vi "Main.vi"() -> ()   [LabVIEW 2017]
uses:
  TypeDefs/StateMachnie_States.ctl
  <vilib>/ni845x/ni845x.llb/ni845xI2cConfiguration.ctl
  <vilib>/ni845x/ni845x.llb/ni845xControl.ctl
  TypeDefs/AD5933_Config.ctl
  TypeDefs/MeasurementConfig.ctl
  TypeDefs/MeasurementRawData.ctl
  TypeDefs/AD5933_OperationState.ctl
  <vilib>/ni845x/ni845x.llb/NI-845x I2C Close Configuration Reference.vi
  <vilib>/ni845x/ni845x.llb/NI-845x Close Device Reference.vi
  GlobalVariables/Delimiter.vi
  GlobalVariables/MeasurementCluster.vi
  <vilib>/imath/engines/lvmath2/RunTimeEngine/Managers/WorkSpace/UID Generator.vi
  <vilib>/imath/engines/lvmath2/RunTimeEngine/ArithmeticOperatorToken/NIMS_ArithmeticOperator_plus.vi
  <instcachedir>/0/NIMS_ArithmeticOperator_plus_9255C7DA94A9479C92F91DC2DA9A664F.lvgen/NIMS_ArithmeticOperator_plus_9255C7DA94A9479C92F91DC2DA9A664F_004.vi
  <vilib>/imathl/engines/lvmath/Functions/Error Handling/Create Error.vi
  <vilib>/imath/engines/lvmath2/RunTimeEngine/ArithmeticOperatorToken/NIMS_ArithmeticOperator_rightdiv.vi
  <instcachedir>/0/NIMS_ArithmeticOperator_rightdiv_EFA95513F40C4B3084B27C9DE6D5A167.lvgen/NIMS_ArithmeticOperator_rightdiv_EFA95513F40C4B3084B27C9DE6D5A167_005.vi
  <vilib>/imath/engines/lvmath2/RunTimeEngine/RunTimeType/NIMS_RunTimeType_From StrictType (excl LVString).vi
  <instcachedir>/0/NIMS_RunTimeType_From StrictType (excl LVString)_1019F277F0A747EDBCA0F6C52CA54500.lvgen/NIMS_RunTimeType_From StrictType (excl LVString)_1019F277F0A747EDBCA0F6C52CA54500_000.vi
  <vilib>/imath/engines/lvmath2/RunTimeEngine/LocalVariableDefStatement/MC_LocalVariableDefStatement_Display.vi
  <vilib>/imath/engines/lvmath2/RunTimeEngine/Managers/SymbolTable/Clear UID.vi
  <vilib>/imath/engines/lvmath2/RunTimeEngine/NodeEndStatement/NIMS_NodeEndStatement_Output.vi
  <instcachedir>/0/NIMS_NodeEndStatement_Output_53EC0D466D134D7ABD903AC30B43404B.lvgen/NIMS_NodeEndStatement_Output_53EC0D466D134D7ABD903AC30B43404B_005.vi
  <vilib>/imath/engines/lvmath2/RunTimeEngine/ErrorHandling/NIMS_Finalize Error.vi
  <vilib>/imath/engines/lvmath2/RunTimeEngine/Managers/SymbolTable/NIMS_WorkSpace.lvlib
panel:
  out "|Z|,phi vs Time (old)":cluster{"X":dbl, "Y":dbl, "X 2":dbl}[](graph)
  out "Temperature vs Time (old)":cluster{"x-y":dbl, "Temperature":dbl}[](graph)
  out "Real,Imag vs Frequency (old)":cluster{"X":dbl, "Y":dbl, "X 2":dbl}[](graph)
  out "Measurement Indicator":bool
  out "|Z|,phi vs Frequency (old)":cluster{dbl, "Impedance":dbl, "Phase":dbl}[](graph)
  in  "Calibrate":bool
  in  "Ref. Resistor":dbl=100000.0 format="%#_13p"
  in  "Start":bool
  in  "Set Configuration":bool
  in  "Stop Measurement":bool
  out "Next measurement":dbl
  in  "Stop Updating Frequeny Plot":bool
  in  "Tab Control":T1(tab)
  out "|Z|,phi vs Frequency":cluster{dbl, "Impedance":dbl, "Phase":dbl}[](graph) caption="XY Graph"
  out "Real,Imag vs Frequency":cluster{dbl, "Impedance":dbl, "Phase":dbl}[](graph) caption="XY Graph"
  out "Temperature vs Time":cluster{"x-y":dbl, "Temperature":dbl}[](graph) caption="XY Graph"
  in  "Frequency [Hz]":dbl(slide) min=5000.0 max=100000.0 step=2500.0 scale=5000.0..100000.0 scale format="%#_6p"
  out "|Z|,phi vs Time":cluster{dbl, "Impedance":dbl, "Phase":dbl}[](graph) caption="XY Graph"
  # "FEHLER Suche:\n- Bei Messung mit 100k Widerstand\n    - Hohe schwankungen zwischen Inf und 0 (Magnitde)\n    - Wenn dann ist Imag Wert sehr hoch, Real recht klein !?!\n       - Sollte umgekehrt Re hocher Leitwert, Im geringer Wert"
  # "Mehrere Werte mitteln ?\nGain Faktor Messen\nAbspeichern noch nicht implementiert!"
  # "[s]"
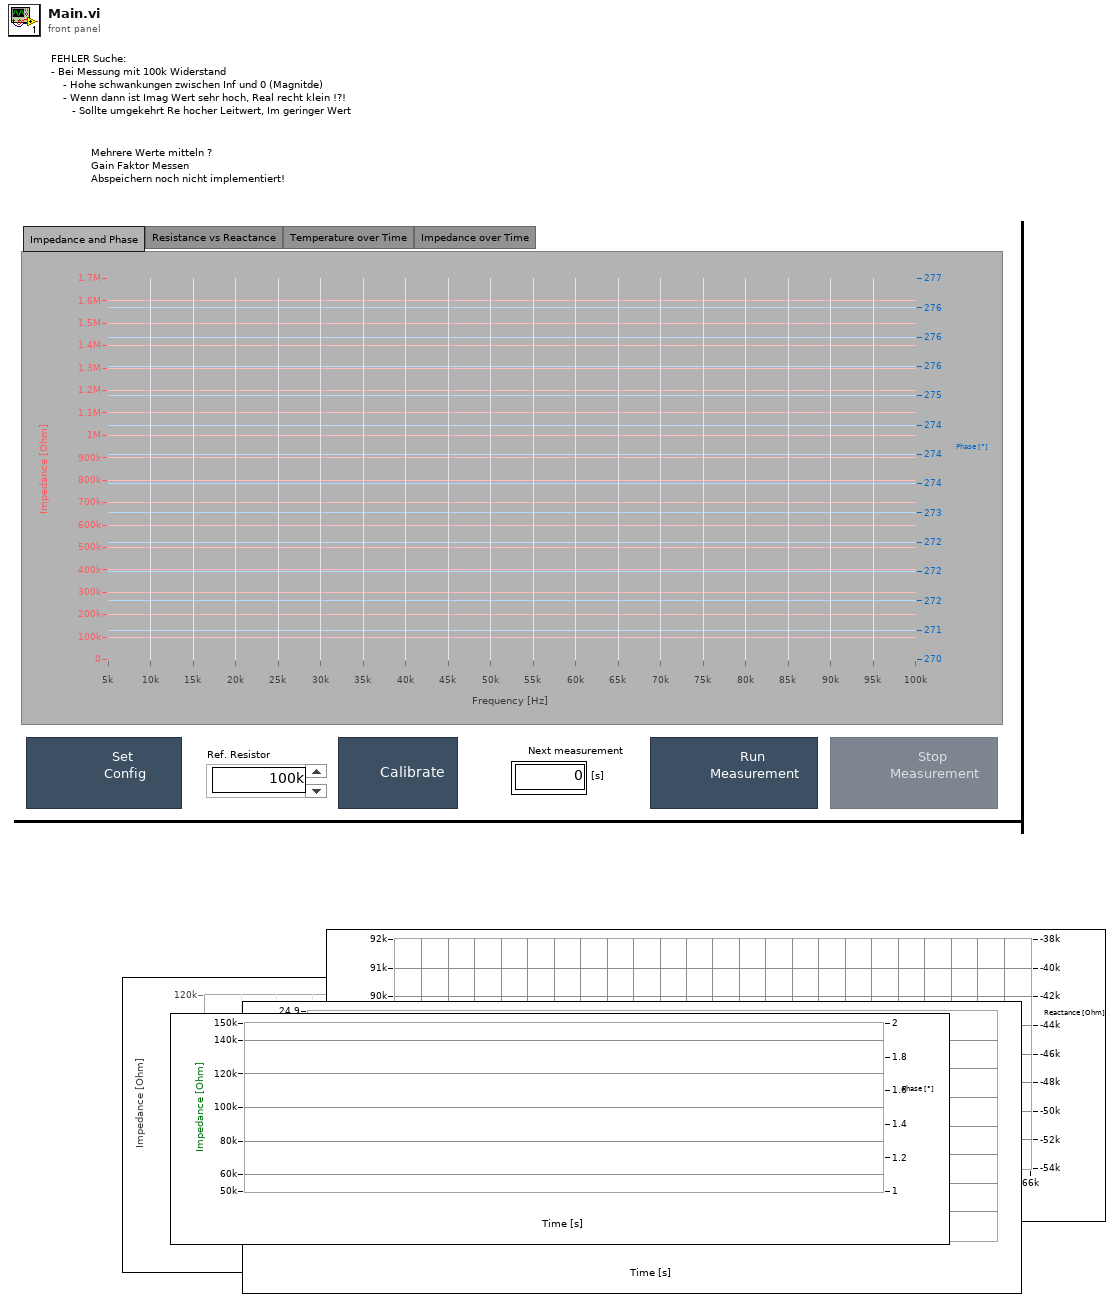
[diagram p1: front panel]
types:
  T1 = enum32{"Impedance and Phase", "Resistance vs Reactance", "Temperature over Time", "Impedance over Time"}
  T2 = typedef "MeasurementRawData.ctl" = cluster{"Temperature":dbl, "R Array":dbl[], "I Array":dbl[], "Measurement Time":timestamp, "GainFactor Array":dbl[], "SystemPhase":dbl[]}
  T3 = cluster{"ConfigRegister (0x80)":u8, "Start Time":timestamp}
  T4 = typedef "MeasurementConfig.ctl" = cluster{"File Path":path, "Sampling Rate [s]":dbl, "SaveMeas":bool, "Frequencies":dbl[], "refnum out":refnum<file>}
  T5 = typedef "AD5933_Config.ctl" = cluster{"Start Frequency / Hz":dbl, "Frequency Increment / Hz":dbl, "Number of Increments / #":u16, "Number of Setting Time Cycles / # ":u16, "Exitation Voltage":enum8{"2V", "200mV", "400mV", "1V"}, "PGA Gain":enum8{"5x", "1x"}}
  T6 = typedef "ni845xI2cConfiguration.ctl" = refnum<k20>
  T7 = typedef "ni845xControl.ctl" = refnum<k21>
  T8 = typedef "StateMachnie_States.ctl" = enum16{"Init", "Wait for Instructions", "Set Configuration", "Calibrate", "Init Measurement", "Do Measurement", "Proceed Measurement and Wait", "Stop Measurement", "Exit"}
  T9 = enum8{"Enabled", "Disabled", "Disabled and Grayed Out"}
  T10 = cluster{"Impedance Array":dbl[][], "Phase Array":dbl[][], "Time Array":dbl[], "Temperature Array":dbl[]}
  T11 = cluster{"Impedance Matrix":dbl[][], "Phase Matrix":dbl[][], "Time Array":dbl[], "Temperature Array":dbl[]}
  T12 = typedef "AD5933_OperationState.ctl" = u8
  T13 = cluster{"i2c configuration out":T6, "Refnum out":T7}
  T14 = typedef "AD5933_FreqSweepConfigRegisterArray.ctl" = u8[]
  T15 = cluster{"x-y":dbl, "Impedance":dbl, "Phase":dbl}[]
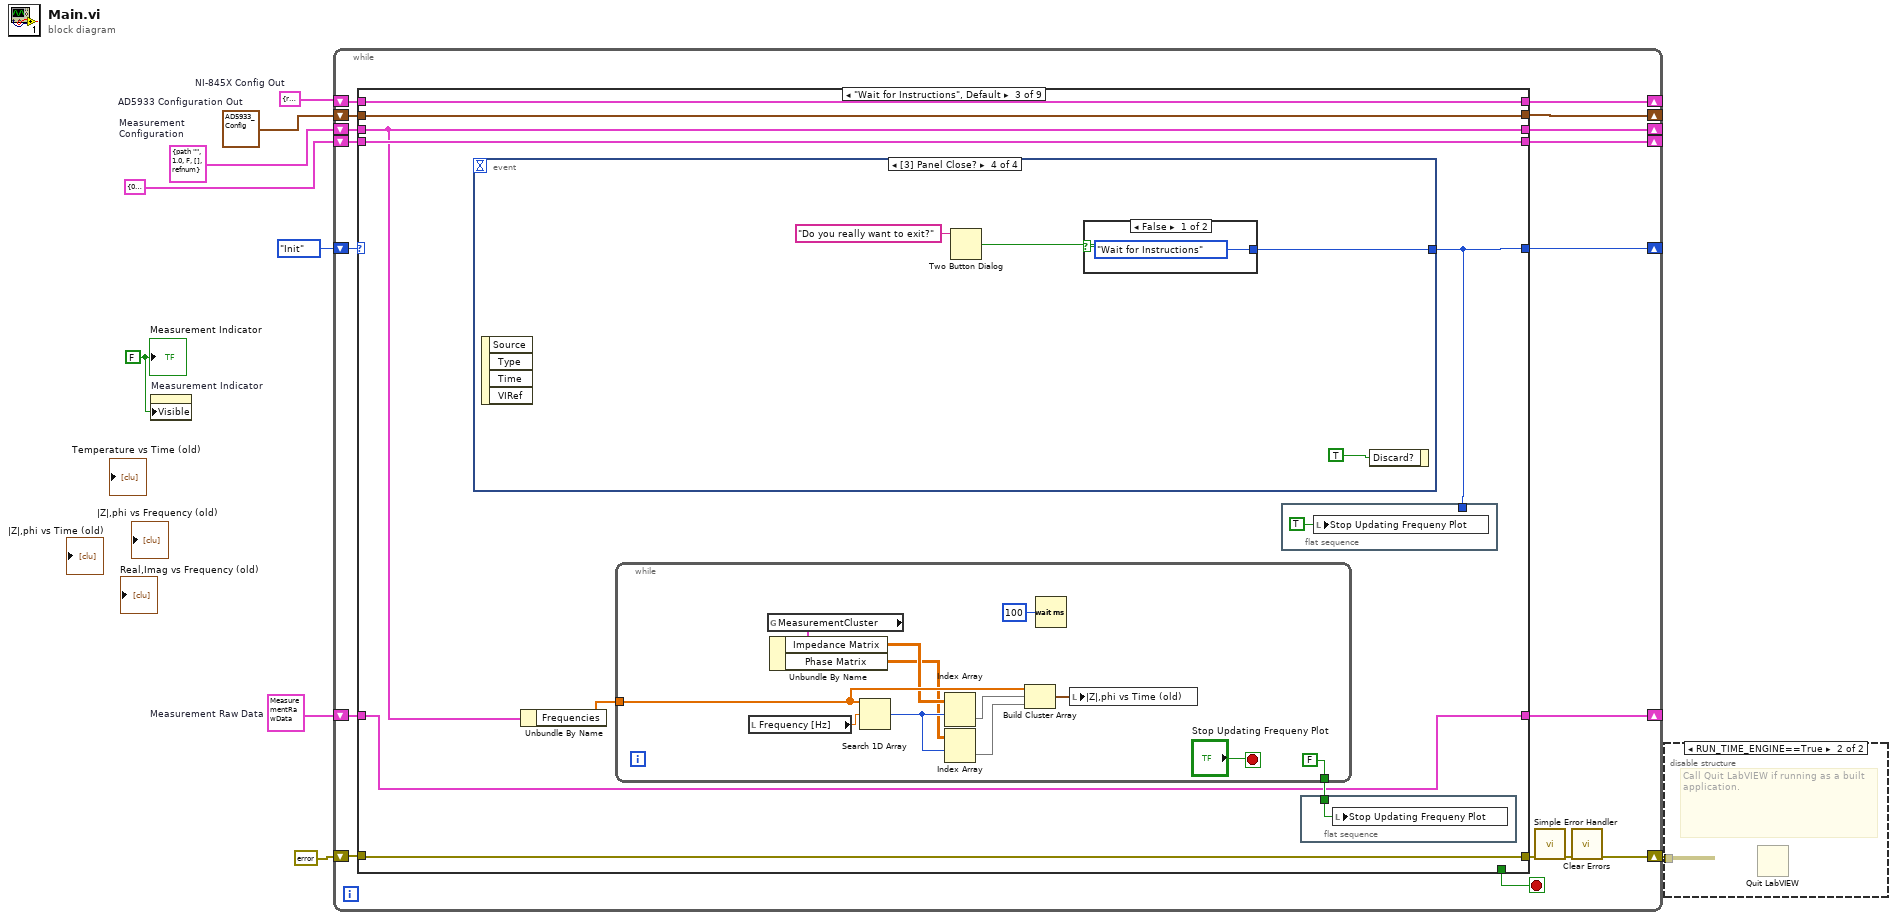
[diagram p0: block diagram]
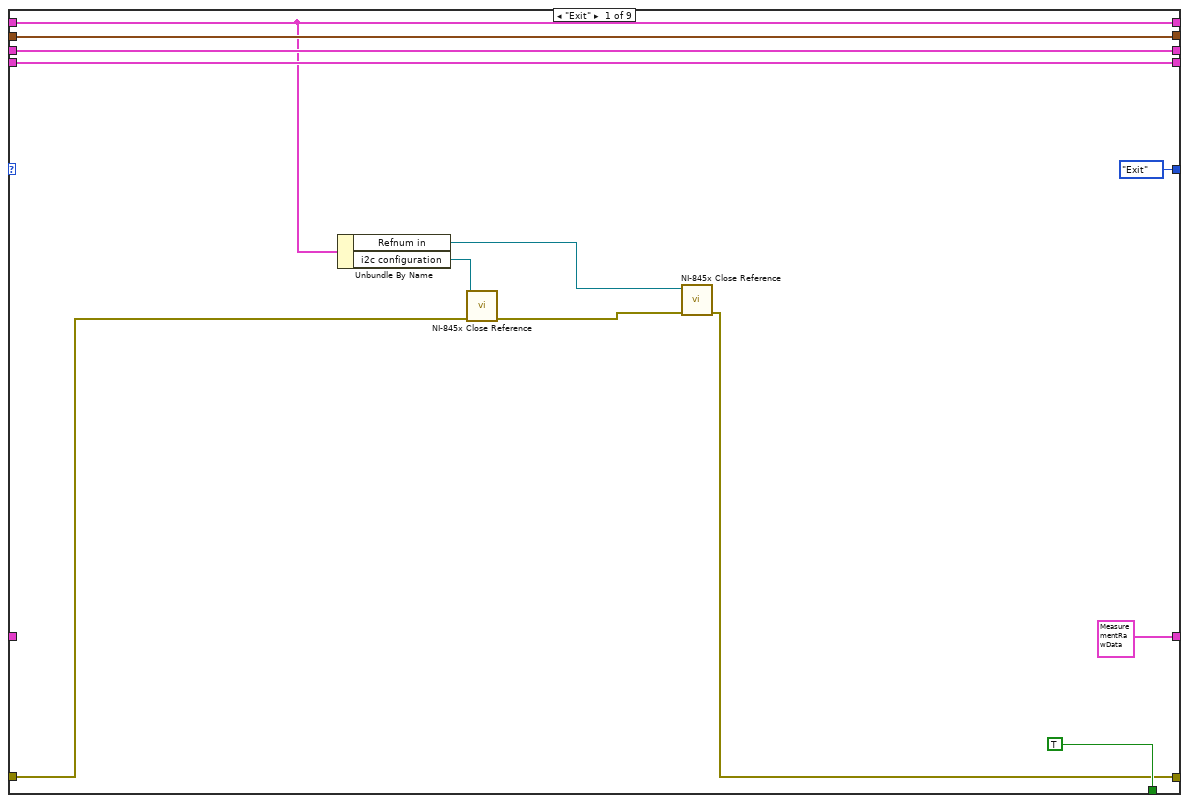
[diagram p3: hidden frame]
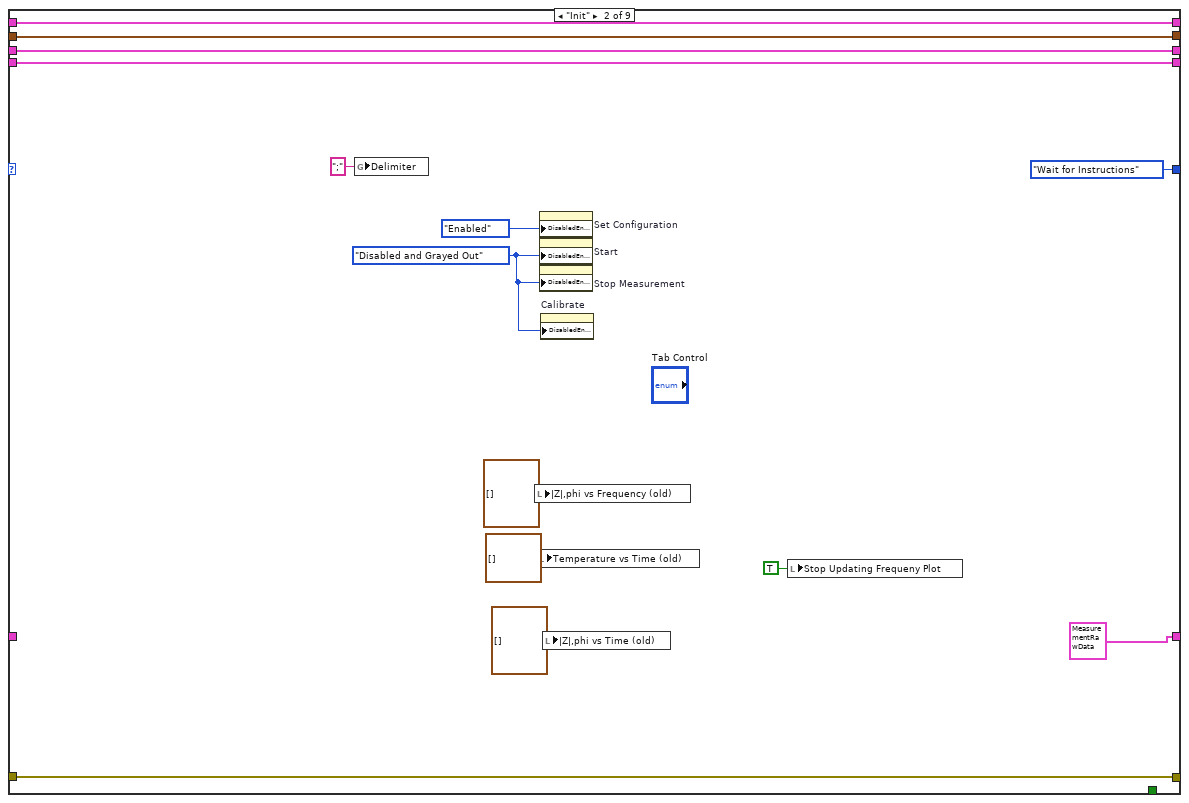
[diagram p4: hidden frame]
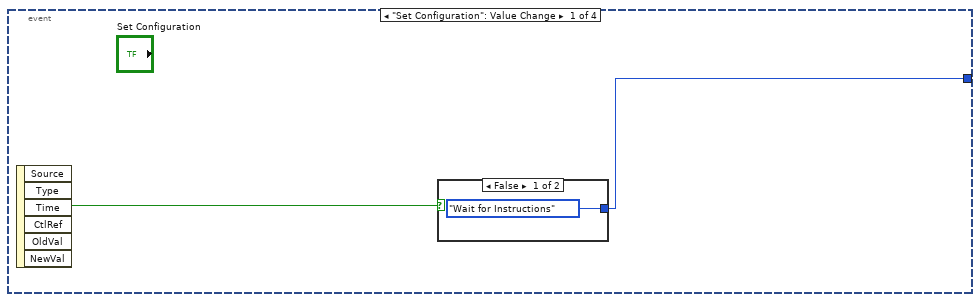
[diagram p5: hidden frame]
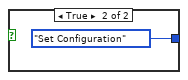
[diagram p6: hidden frame]
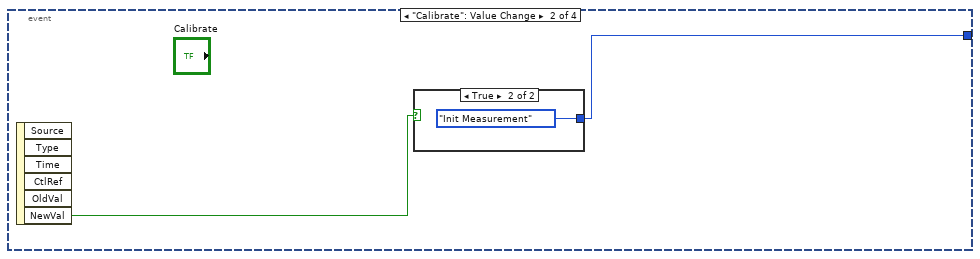
[diagram p7: hidden frame]
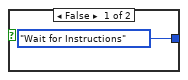
[diagram p8: hidden frame]
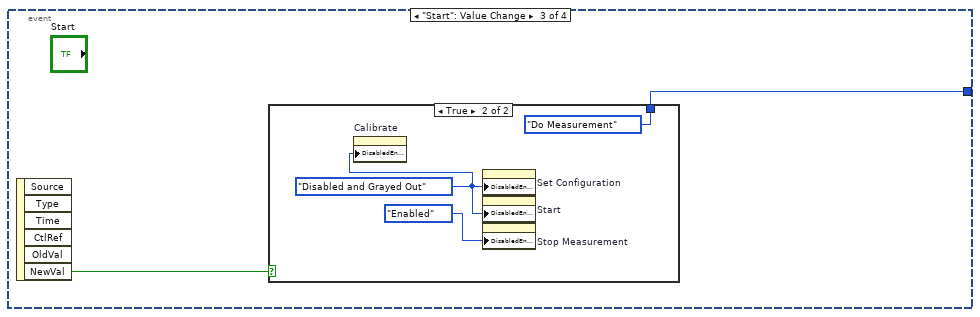
[diagram p9: hidden frame]
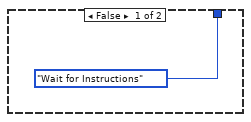
[diagram p10: hidden frame]
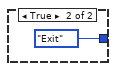
[diagram p11: hidden frame]
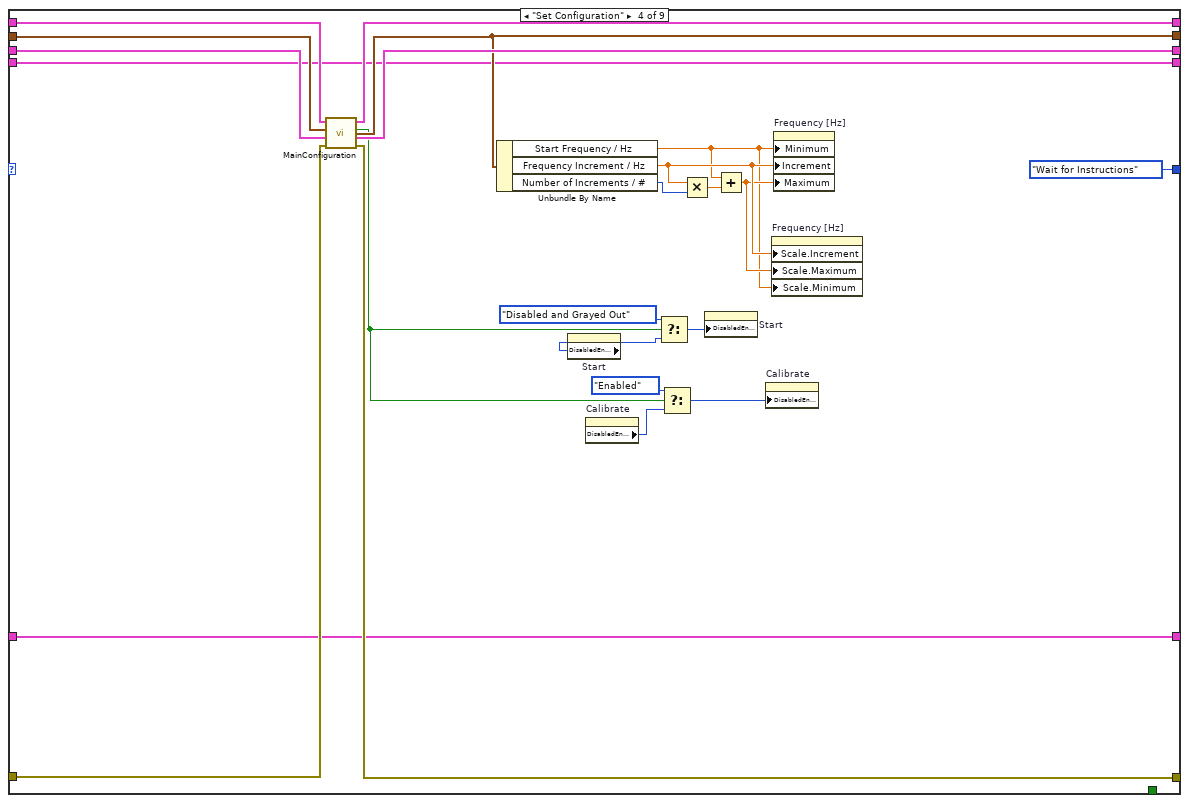
[diagram p12: hidden frame]
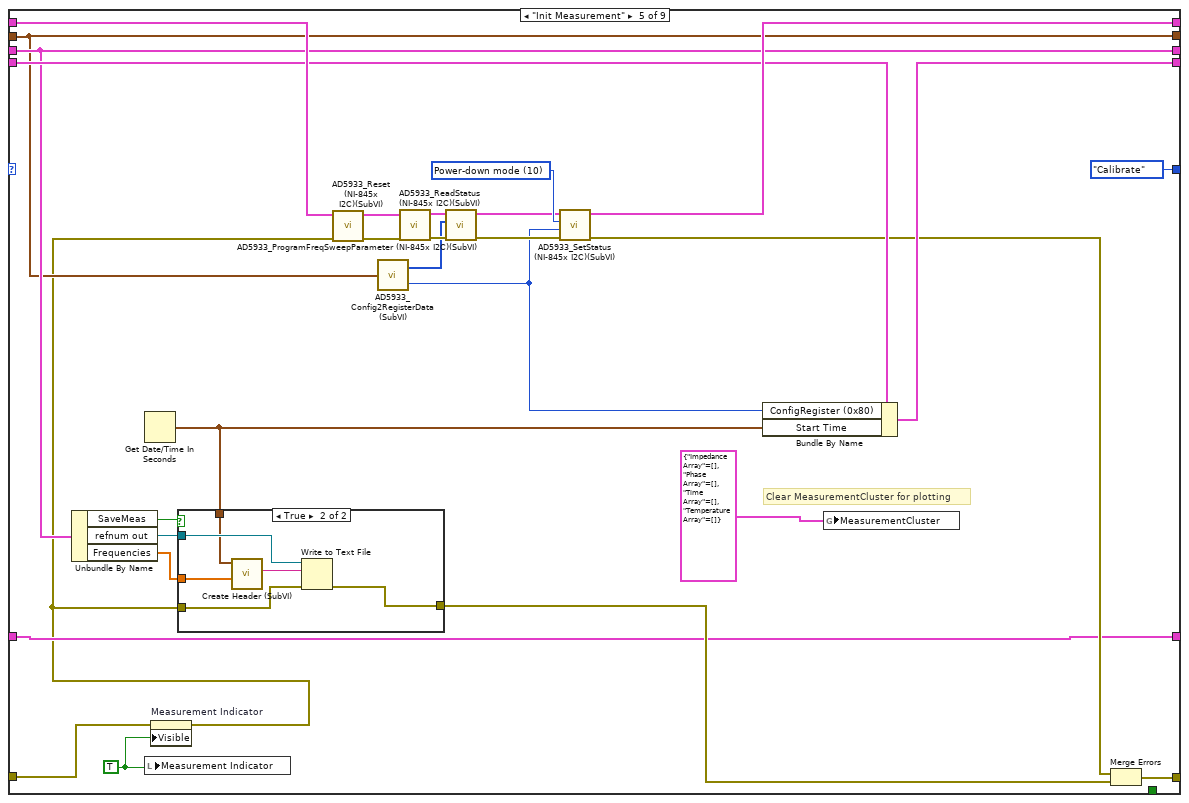
[diagram p13: hidden frame]
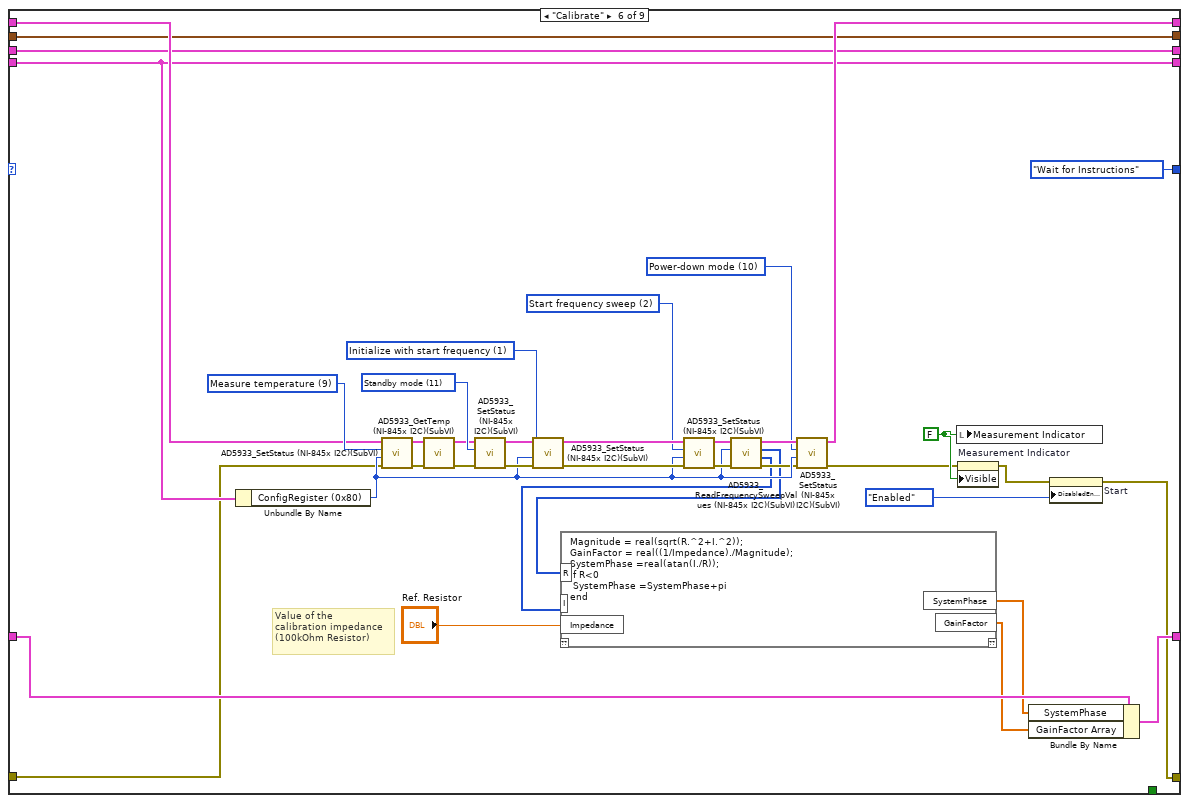
[diagram p15: hidden frame]
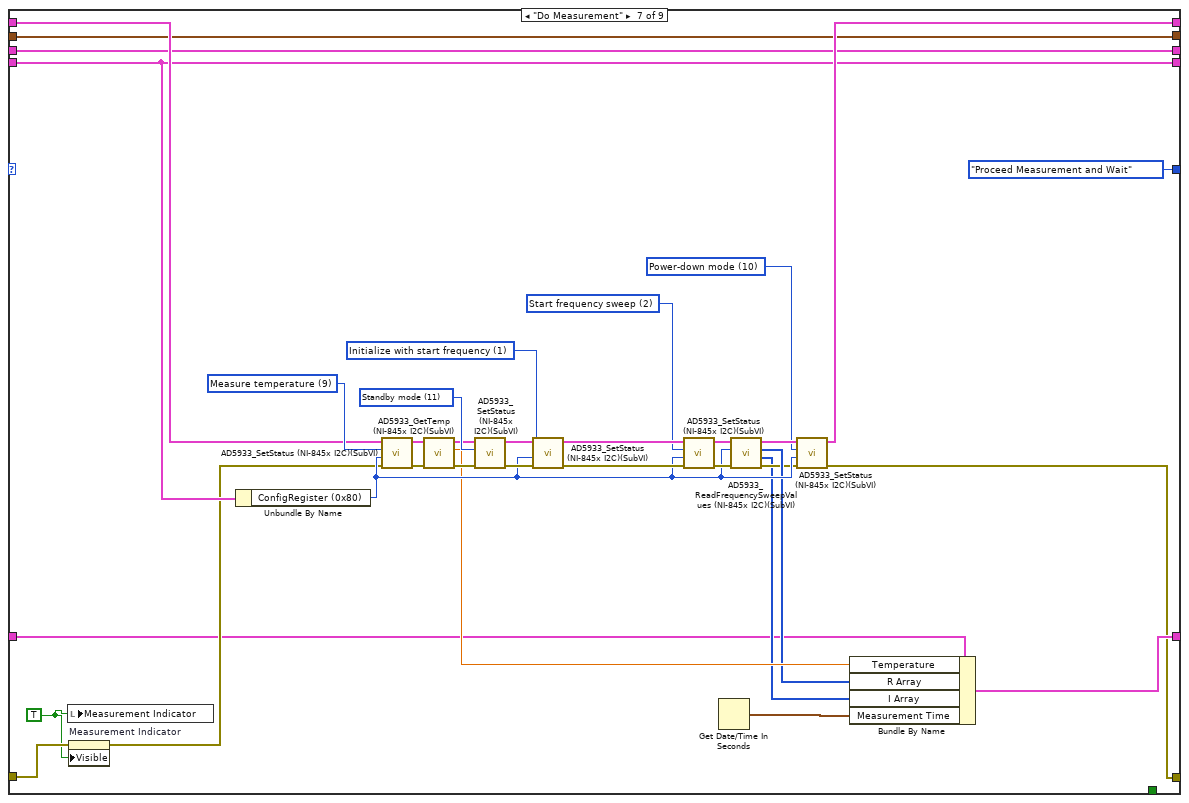
[diagram p16: hidden frame]
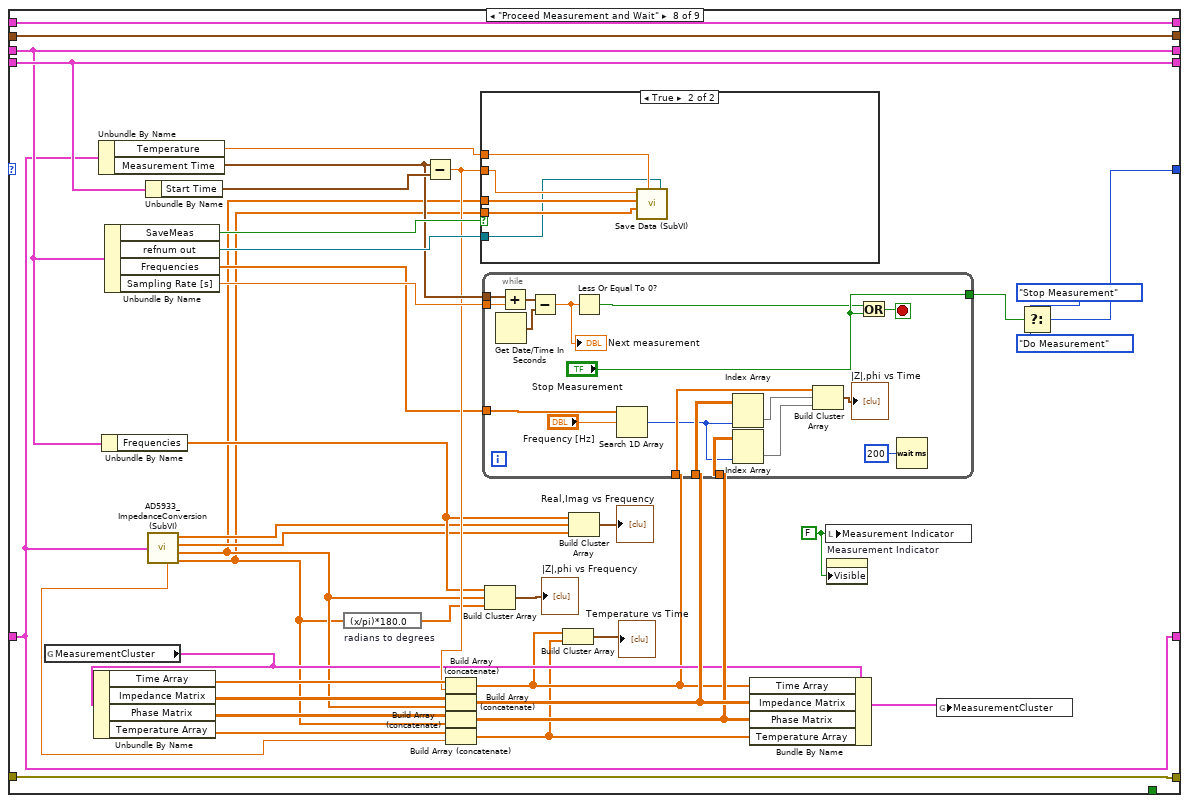
[diagram p17: hidden frame]
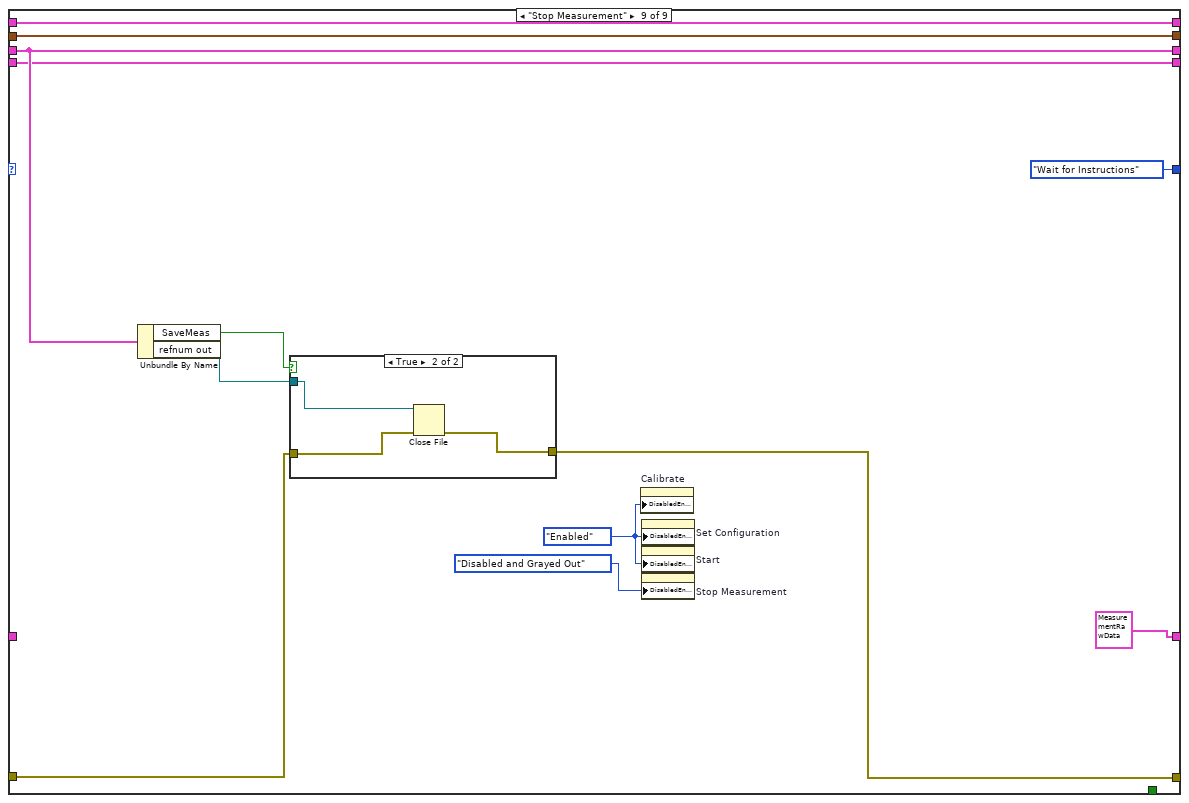
[diagram p19: hidden frame]
diagram:
  w1 = FALSE ("Measurement Indicator")
  w3 = T2 {"Temperature"=0.0, "R Array"=[], "I Array"=[], "Measurement Time"=timestamp(0 s since 1904-01-01), "GainFactor Array"=[], "SystemPhase"=[]}  # Measurement Raw Data
  w5 = T4 {"File Path"=path "", "Sampling Rate [s]"=1.0, "SaveMeas"=FALSE, "Frequencies"=[], "refnum out"=refnum}  # Measurement  Configuration
  w6 = T5 {"Start Frequency / Hz"=55000.0, "Frequency Increment / Hz"=1000.0, "Number of Increments / #"=9, "Number of Setting Time Cycles / # "=2044, "Exitation Voltage"=enum."1V", "PGA Gain"=enum."5x"}  # AD5933 Configuration Out
  w7 = cluster{"i2c configuration":T6, "Refnum in":T7} {"i2c configuration"=refnum, "Refnum in"="USB0::0x3923::0x7514::019441AA::RAW"}  # NI-845X Config Out
  n1 = property on="Measurement Indicator" class="Bool"("Visible"=w1) -> ()  [unwired: 2 in, 2 out]
  n2 = while {
    shift-right: [w25] -> _
    shift-left: StateMachnie_States."Init" -> [w26]
    shift-right: [w11] -> w2
    shift-left: errorcluster {"status"=FALSE, "code"=0, "source"=""} ("error out") -> [w24]
    shift-right: [w23] -> _
    shift-left: w7 -> [w20]
    shift-right: [w22] -> _
    shift-left: w6 -> [w21]
    shift-right: [w18] -> _
    shift-left: w5 -> [w19]
    shift-right: [w16] -> _
    shift-left: T3 {"ConfigRegister (0x80)"=0, "Start Time"=timestamp(0 s since 1904-01-01)} -> [w17]
    shift-right: [w15] -> _
    shift-left: w3 -> [w10]
    stop <- w14 stop-if-true
    n3 = case shown="\"Wait for Instructions\", Default" w26 {
      tunnel: [StateMachnie_States."Exit" StateMachnie_States."Wait for Instructions" w56 StateMachnie_States."Wait for Instructions" StateMachnie_States."Calibrate" StateMachnie_States."Wait for Instructions" StateMachnie_States."Proceed Measurement and Wait" w367 StateMachnie_States."Wait for Instructions"] -> w25
      tunnel: w24 -> [w29 w51 w54 w118 w120 w157 w309 w360 w412]
      tunnel: [w28 w51 w54 w117 w128 w155 w310 w360 w403] -> w12
      tunnel: [w27 w50 w60 w116 w139 w179 w328 w377 w411] -> w23
      tunnel: [w36 w49 w59 w111 w130 w170 w315 w376 w410] -> w22
      tunnel: w21 -> [w36 w49 w59 w113 w130 w170 w315 w376 w410]
      tunnel: w20 -> [w27 w50 w60 w114 w141 w174 w323 w377 w411]
      tunnel: w19 -> [w35 w48 w58 w115 w133 w169 w314 w366 w409]
      tunnel: [w35 w48 w58 w112 w133 w169 w314 w366 w409] -> w18
      tunnel: w17 -> [w34 w47 w61 w104 w135 w168 w313 w375 w408]
      tunnel: [w34 w47 w61 w104 w134 w168 w313 w375 w408] -> w16
      tunnel: w10 -> [_ _ w53 w103 w122 w162 w306 w350 _]
      tunnel: [T2 {"Temperature"=0.0, "R Array"=[], "I Array"=[], "Measurement Time"=timestamp(0 s since 1904-01-01), "GainFactor Array"=[], "SystemPhase"=[]} ("Measurement Raw Data") T2 {"Temperature"=0.0, "R Array"=[], "I Array"=[], "Measurement Time"=timestamp(0 s since 1904-01-01), "GainFactor Array"=[], "SystemPhase"=[]} ("Measurement Raw Data") w53 w103 w122 w161 w316 w350 T2 {"Temperature"=0.0, "R Array"=[], "I Array"=[], "Measurement Time"=timestamp(0 s since 1904-01-01), "GainFactor Array"=[], "SystemPhase"=[]} ("Measurement Raw Data")] -> w15
      tunnel: [TRUE _ _ _ _ _ _ _ _] -> w14
      frame "Exit" {
        n4 = Unbundle By Name(w27) -> ("Refnum in"=w31:T7, "i2c configuration"=w32:T6)
        n5 = call-poly <vilib>:"NI-845x Close Reference.vi"("error in (no error)"=w29, "i2c configuration"=w32) -> ("error out"=w30:errorcluster)  [unwired: 9 in]
        n6 = call-poly <vilib>:"NI-845x Close Reference.vi"("error in (no error)"=w30, "device reference"=w31) -> ("error out"=w28:errorcluster)  [unwired: 9 in]
      }
      frame "Init" {
        w41 = T9."Disabled and Grayed Out" ("Disabled")
        n7 = global write "Delimiter.vi" "Delimiter"(";" ("Delimiter")) -> ()
        n8 = local write "|Z|,phi vs Frequency (old)"(cluster{"X":dbl, "Y":dbl, "X 2":dbl}[] [] ("|Z|,phi vs Frequency")) -> ()
        n9 = local write "Temperature vs Time (old)"(cluster{"x-y":dbl, "Temperature":dbl}[] [] ("Temperature vs Time")) -> ()
        n10 = property on="Set Configuration" class="Bool"("DisabledEnum"=T9."Enabled" ("Disabled")) -> ()  [unwired: 2 in, 2 out]
        n11 = property on="Start" class="Bool"("DisabledEnum"=w41) -> ()  [unwired: 2 in, 2 out]
        n12 = property on="Stop Measurement" class="Bool"("DisabledEnum"=w41) -> ()  [unwired: 2 in, 2 out]
        n13 = property on="Calibrate" class="Bool"("DisabledEnum"=w41) -> ()  [unwired: 2 in, 2 out]
        n14 = local write "|Z|,phi vs Time (old)"(cluster{"X":dbl, "Y":dbl, "X 2":dbl}[] [] ("|Z|,phi vs Time")) -> ()
        n15 = local write "Stop Updating Frequeny Plot"(TRUE ("Stop Updating Frequeny Plot")) -> ()
      }
      frame "Wait for Instructions", Default {
        n16 = event shown="[3] Panel Close?" {
          selector: _ -> [_ _ _ _]
          dyn-events: _ -> [_ _ _ _]
          timeout: _ -> [_ _ _ _]
          tunnel: [w76 w81 w84 w91] -> w56
          event "Set Configuration": Value Change {
            n17 = event-data() -> ("NewVal"=w77:bool)  [unwired: 1 in, 5 out]
            n18 = case shown="False" w77 {
              tunnel: [StateMachnie_States."Wait for Instructions" StateMachnie_States."Set Configuration"] -> w76
              frame False {
              }
              frame True {
              }
            }
          }
          event "Calibrate": Value Change {
            n19 = event-data() -> ("NewVal"=w80:bool)  [unwired: 1 in, 5 out]
            n20 = case shown="True" w80 {
              tunnel: [StateMachnie_States."Wait for Instructions" StateMachnie_States."Init Measurement"] -> w81
              frame False {
              }
              frame True {
              }
            }
          }
          event "Start": Value Change {
            n21 = event-data() -> ("NewVal"=w85:bool)  [unwired: 1 in, 5 out]
            n22 = case shown="True" w85 {
              tunnel: [StateMachnie_States."Wait for Instructions" StateMachnie_States."Do Measurement"] -> w84
              frame False {
              }
              frame True {
                w87 = T9."Disabled and Grayed Out" ("Disabled")
                n23 = property on="Calibrate" class="Bool"("DisabledEnum"=w87) -> ()  [unwired: 2 in, 2 out]
                n24 = property on="Set Configuration" class="Bool"("DisabledEnum"=w87) -> ()  [unwired: 2 in, 2 out]
                n25 = property on="Start" class="Bool"("DisabledEnum"=w87) -> ()  [unwired: 2 in, 2 out]
                n26 = property on="Stop Measurement" class="Bool"("DisabledEnum"=T9."Enabled" ("Disabled")) -> ()  [unwired: 2 in, 2 out]
              }
            }
          }
          event Panel Close? {
            n27 = event-data() -> ()  [unwired: 1 in, 4 out]
            n28 = Two Button Dialog(message="Do you really want to exit?") -> (T button?=w90:bool)  [unwired: 2 in]
            n29 = case shown="False" w90 {
              tunnel: [StateMachnie_States."Wait for Instructions" StateMachnie_States."Exit"] -> w91
              frame False {
              }
              frame True {
              }
            }
            n30 = event-data("Discard?"=TRUE) -> ()  [unwired: 1 in, 1 out]
          }
        }
        n31 = Unbundle By Name(w58) -> ("Frequencies"=w57:dbl[])
        n32 = while {
          tunnel: w57 -> [w75]
          tunnel: [FALSE ("Stop Updating Frequeny Plot")] -> w55
          stop <- "Stop Updating Frequeny Plot" stop-if-true
          n33 = local read "Frequency [Hz]"() -> (w68:dbl)
          n34 = global read "MeasurementCluster.vi" "MeasurementCluster"() -> (w71:T11)
          n35 = Unbundle By Name(w71) -> ("Impedance Matrix"=w70:dbl[][], "Phase Matrix"=w69:dbl[][])
          n36 = Search 1D Array(1D array=w75, element=w68) -> (index of element=w74:i32)  [unwired: 1 in]
          n37 = Index Array(array=w70, index (row)=w74) -> (element=w73:dbl[])  [unwired: 1 in]
          n38 = Index Array(array=w69, index (row)=w74) -> (element=w72:dbl[])  [unwired: 1 in]
          n39 = Build Cluster Array(w75, w73, w72) -> (w65:cluster{dbl, dbl, dbl}[])
          n40 = Wait (ms)(milliseconds to wait=u32 100) -> ()  [unwired: 1 out]
          n41 = local write "|Z|,phi vs Time (old)"(w65) -> ()
        }
        n42 = flat-sequence {
          tunnel: w56 -> [_]
          frame #0 {
            n43 = local write "Stop Updating Frequeny Plot"(TRUE ("Stop Updating Frequeny Plot")) -> ()
          }
        }
        n44 = flat-sequence {
          tunnel: w55 -> [w62]
          frame #0 {
            n45 = local write "Stop Updating Frequeny Plot"(w62) -> ()
          }
        }
      }
      frame "Set Configuration" {
        n46 = call "MainConfiguration.vi"("NI-845X Config"=w114, "AD5933 Configuration"=w113, "Measurement \nConfiguration"=w115, "error in (no error)"=w118) -> ("AD5933 Configuration Out"=w111:T5, "NI-845X Config Out"=w116:cluster{"i2c configuration":T6, "Refnum in":T7}, "New Setup"=w99:bool, "Measurement \nConfiguration out"=w112:T4, "error out"=w117:errorcluster)
        n47 = Unbundle By Name(w111) -> ("Start Frequency / Hz"=w106:dbl, "Frequency Increment / Hz"=w108:dbl, "Number of Increments / #"=w110:u16)
        n48 = property on="Start" class="Bool"() -> ("DisabledEnum"=w96:T9)  [unwired: 2 in, 2 out]
        n49 = property on="Calibrate" class="Bool"() -> ("DisabledEnum"=w97:T9)  [unwired: 2 in, 2 out]
        n50 = Select(t=T9."Disabled and Grayed Out" ("Disabled"), s=w99, f=w96) -> (s? t:f=w102:T9)
        n51 = Select(t=T9."Enabled" ("Disabled"), s=w99, f=w97) -> (s? t:f=w98:T9)
        n52 = Multiply(x=w108, y=w110) -> (x*y=w109:dbl)
        n53 = property on="Start" class="Bool"("DisabledEnum"=w102) -> ()  [unwired: 2 in, 2 out]
        n54 = Add(x=w106, y=w109) -> (x+y=w107:dbl)
        n55 = property on="Calibrate" class="Bool"("DisabledEnum"=w98) -> ()  [unwired: 2 in, 2 out]
        n56 = property on="Frequency [Hz]" class="Slide (strict)"("Scale.Increment"=w108, "Scale.Maximum"=w107, "Scale.Minimum"=w106) -> ()  [unwired: 2 in, 2 out]
        n57 = property on="Frequency [Hz]" class="Slide (strict)"("Minimum"=w106, "Increment"=w108, "Maximum"=w107) -> ()  [unwired: 2 in, 2 out]
      }
      frame "Init Measurement" {
        w121 = TRUE ("Visible")
        w140 = T12 10 items=["Initialize with start frequency"=1, "Start frequency sweep"=2, "Increment frequency"=3, "Repeat frequency"=4, "Measure temperature"=9, "Power-down mode"=10, "Standby mode"=11] ("ControlRegisterStates(D15-D12)")
        # "Clear MeasurementCluster for plotting"
        n58 = Unbundle By Name(w133) -> ("SaveMeas"=w132:bool, "refnum out"=w131:refnum<file>, "Frequencies"=w126:dbl[])
        n59 = Get Date/Time In Seconds() -> (seconds since 1Jan1904=w125:timestamp)
        n60 = local write "Measurement Indicator"(w121) -> ()
        n61 = property on="Measurement Indicator" class="Bool"(error in=w120, "Visible"=w121) -> (error out=w119:errorcluster)  [unwired: 1 in, 1 out]
        n62 = case shown="True" w132 {
          tunnel: w131 -> [_ w151]
          tunnel: w119 -> [w147 w150]
          tunnel: [w147 w152] -> w129
          tunnel: w126 -> [_ w149]
          tunnel: w125 -> [_ w148]
          frame False {
          }
          frame True {
            n63 = call "Create Header (SubVI).vi"("Frequencies"=w149, "current time"=w148) -> ("Header"=w153:string)  [unwired: 9 in]
            n64 = Write to Text File(file (use dialog)=w151, text=w153, error in=w150) -> (error out=w152:errorcluster)  [unwired: 1 in, 2 out]
          }
        }
        n65 = call "AD5933_Reset (NI-845x I2C)(SubVI).vi"("error in"=w119, "NI-845x Config for I2C (in)"=w141) -> ("error out"=w143:errorcluster, "NI-845x Config for I2C (out)"=w144:T13)  [unwired: 7 in]
        n66 = call "AD5933_Config2RegisterData (SubVI).vi"("AD5933 Configuration"=w130) -> ("FrequencySweepConfigArray (Reg 0x82-0x8B)"=w142:T14, "ConfigRegister (0x80)"=w136:u8)
        n67 = call "AD5933_ReadStatus (NI-845x I2C)(SubVI).vi"("error in"=w143, "NI-845x Config for I2C (in)"=w144) -> ("error out"=w146:errorcluster, "NI-845x Config for I2C (out)"=w145:T13)  [unwired: 6 in, 1 out]
        n68 = call "AD5933_ProgramFreqSweepParameter (NI-845x I2C)(SubVI).vi"("error in"=w146, "FrequencySweepConfigArray (Reg 0x82-0x8B)"=w142, "NI-845x Config for I2C (in)"=w145) -> ("error out"=w138:errorcluster, "NI-845x Config for I2C (out)"=w137:T13)  [unwired: 6 in]
        n69 = call "AD5933_SetStatus (NI-845x I2C)(SubVI).vi"("error in"=w138, "ConfigRegister (0x80)"=w136, "ControlRegisterStates(D15-D12)"=w140, "NI-845x Config for I2C (in)"=w137) -> ("error out"=w127:errorcluster, "NI-845x Config for I2C (out)"=w139:T13)  [unwired: 5 in]
        n70 = Bundle By Name(cluster=w135, "ConfigRegister (0x80)"=w136, "Start Time"=w125) -> (w134:T3)
        n71 = global write "MeasurementCluster.vi" "MeasurementCluster"(T10 {"Impedance Array"=[], "Phase Array"=[], "Time Array"=[], "Temperature Array"=[]} ("MeasurementCluster")) -> ()
        n72 = Merge Errors(w127, w129) -> (w128:errorcluster)
      }
      frame "Calibrate" {
        w166 = FALSE ("Visible")
        w176 = T12 9 items=["Initialize with start frequency"=1, "Start frequency sweep"=2, "Increment frequency"=3, "Repeat frequency"=4, "Measure temperature"=9, "Power-down mode"=10, "Standby mode"=11] ("ControlRegisterStates(D15-D12)")
        w186 = T12 2 items=["Initialize with start frequency"=1, "Start frequency sweep"=2, "Increment frequency"=3, "Repeat frequency"=4, "Measure temperature"=9, "Power-down mode"=10, "Standby mode"=11] ("ControlRegisterStates(D15-D12)")
        w182 = T12 11 items=["Initialize with start frequency"=1, "Start frequency sweep"=2, "Increment frequency"=3, "Repeat frequency"=4, "Measure temperature"=9, "Power-down mode"=10, "Standby mode"=11] ("ControlRegisterStates(D15-D12)")
        w180 = T12 10 items=["Initialize with start frequency"=1, "Start frequency sweep"=2, "Increment frequency"=3, "Repeat frequency"=4, "Measure temperature"=9, "Power-down mode"=10, "Standby mode"=11] ("ControlRegisterStates(D15-D12)")
        w188 = T12 1 items=["Initialize with start frequency"=1, "Start frequency sweep"=2, "Increment frequency"=3, "Repeat frequency"=4, "Measure temperature"=9, "Power-down mode"=10, "Standby mode"=11] ("ControlRegisterStates(D15-D12)")
        # "Value of the \ncalibration impedance\n(100kOhm Resistor)"
        n73 = Unbundle By Name(w168) -> ("ConfigRegister (0x80)"=w172:u8)
        n74 = call "AD5933_SetStatus (NI-845x I2C)(SubVI).vi"("error in"=w157, "ConfigRegister (0x80)"=w172, "ControlRegisterStates(D15-D12)"=w176, "NI-845x Config for I2C (in)"=w174) -> ("error out"=w178:errorcluster, "NI-845x Config for I2C (out)"=w177:T13)  [unwired: 5 in]
        n75 = call "AD5933_GetTemp (NI-845x I2C)(SubVI).vi"("error in (no error)"=w178, "NI-845x Config for I2C (out) in"=w177) -> ("error out"=w173:errorcluster, "NI-845x Config for I2C (out) out"=w175:T13)  [unwired: 7 in, 1 out]
        n76 = call "AD5933_SetStatus (NI-845x I2C)(SubVI).vi"("error in"=w173, "ControlRegisterStates(D15-D12)"=w182, "NI-845x Config for I2C (in)"=w175) -> ("error out"=w190:errorcluster, "NI-845x Config for I2C (out)"=w189:T13)  [unwired: 6 in]
        n77 = call "AD5933_SetStatus (NI-845x I2C)(SubVI).vi"("error in"=w190, "ConfigRegister (0x80)"=w172, "ControlRegisterStates(D15-D12)"=w188, "NI-845x Config for I2C (in)"=w189) -> ("error out"=w185:errorcluster, "NI-845x Config for I2C (out)"=w187:T13)  [unwired: 5 in]
        n78 = call "AD5933_SetStatus (NI-845x I2C)(SubVI).vi"("error in"=w185, "ConfigRegister (0x80)"=w172, "ControlRegisterStates(D15-D12)"=w186, "NI-845x Config for I2C (in)"=w187) -> ("error out"=w184:errorcluster, "NI-845x Config for I2C (out)"=w183:T13)  [unwired: 5 in]
        n79 = call "AD5933_ReadFrequencySweepValues (NI-845x I2C)(SubVI).vi"("error in"=w184, "ConfigRegister (0x80)"=w172, "NI-845x Config for I2C (in)"=w183) -> ("error out"=w171:errorcluster, "I Array"=w164:i16[], "R Array"=w165:i16[], "NI-845x Config for I2C (out)"=w181:T13)  [unwired: 4 in]
        n80 = mathscript code="Magnitude = real(sqrt(R.^2+I.^2));\nGainFactor = real((1/Impedance)./Magnitude);\nSystemPhase =real(atan(I./R));\nif R<0\n SystemPhase =SystemPhase+pi\nend"("R"=w165, "I"=w164, "Impedance"="Ref. Resistor") -> ("SystemPhase"=w159:dbl[], "GainFactor"=w160:dbl[])  [unwired: 1 in, 1 out]
        n81 = call "AD5933_SetStatus (NI-845x I2C)(SubVI).vi"("error in"=w171, "ConfigRegister (0x80)"=w172, "ControlRegisterStates(D15-D12)"=w180, "NI-845x Config for I2C (in)"=w181) -> ("error out"=w158:errorcluster, "NI-845x Config for I2C (out)"=w179:T13)  [unwired: 5 in]
        n82 = local write "Measurement Indicator"(w166) -> ()
        n83 = property on="Measurement Indicator" class="Bool"(error in=w158, "Visible"=w166) -> (error out=w156:errorcluster)  [unwired: 1 in, 1 out]
        n84 = Bundle By Name(cluster=w162, "SystemPhase"=w159, "GainFactor Array"=w160) -> (w161:T2)
        n85 = property on="Start" class="Bool"(error in=w156, "DisabledEnum"=T9."Enabled" ("Disabled")) -> (error out=w155:errorcluster)  [unwired: 1 in, 1 out]
      }
      frame "Do Measurement" {
        w307 = TRUE ("Visible")
        w325 = T12 9 items=["Initialize with start frequency"=1, "Start frequency sweep"=2, "Increment frequency"=3, "Repeat frequency"=4, "Measure temperature"=9, "Power-down mode"=10, "Standby mode"=11] ("ControlRegisterStates(D15-D12)")
        w335 = T12 2 items=["Initialize with start frequency"=1, "Start frequency sweep"=2, "Increment frequency"=3, "Repeat frequency"=4, "Measure temperature"=9, "Power-down mode"=10, "Standby mode"=11] ("ControlRegisterStates(D15-D12)")
        w331 = T12 11 items=["Initialize with start frequency"=1, "Start frequency sweep"=2, "Increment frequency"=3, "Repeat frequency"=4, "Measure temperature"=9, "Power-down mode"=10, "Standby mode"=11] ("ControlRegisterStates(D15-D12)")
        w329 = T12 10 items=["Initialize with start frequency"=1, "Start frequency sweep"=2, "Increment frequency"=3, "Repeat frequency"=4, "Measure temperature"=9, "Power-down mode"=10, "Standby mode"=11] ("ControlRegisterStates(D15-D12)")
        w337 = T12 1 items=["Initialize with start frequency"=1, "Start frequency sweep"=2, "Increment frequency"=3, "Repeat frequency"=4, "Measure temperature"=9, "Power-down mode"=10, "Standby mode"=11] ("ControlRegisterStates(D15-D12)")
        n86 = local write "Measurement Indicator"(w307) -> ()
        n87 = property on="Measurement Indicator" class="Bool"(error in=w309, "Visible"=w307) -> (error out=w308:errorcluster)  [unwired: 1 in, 1 out]
        n88 = Unbundle By Name(w313) -> ("ConfigRegister (0x80)"=w321:u8)
        n89 = call "AD5933_SetStatus (NI-845x I2C)(SubVI).vi"("error in"=w308, "ConfigRegister (0x80)"=w321, "ControlRegisterStates(D15-D12)"=w325, "NI-845x Config for I2C (in)"=w323) -> ("error out"=w327:errorcluster, "NI-845x Config for I2C (out)"=w326:T13)  [unwired: 5 in]
        n90 = call "AD5933_GetTemp (NI-845x I2C)(SubVI).vi"("error in (no error)"=w327, "NI-845x Config for I2C (out) in"=w326) -> ("error out"=w322:errorcluster, "Temperature"=w320:dbl, "NI-845x Config for I2C (out) out"=w324:T13)  [unwired: 7 in]
        n91 = call "AD5933_SetStatus (NI-845x I2C)(SubVI).vi"("error in"=w322, "ControlRegisterStates(D15-D12)"=w331, "NI-845x Config for I2C (in)"=w324) -> ("error out"=w339:errorcluster, "NI-845x Config for I2C (out)"=w338:T13)  [unwired: 6 in]
        n92 = call "AD5933_SetStatus (NI-845x I2C)(SubVI).vi"("error in"=w339, "ConfigRegister (0x80)"=w321, "ControlRegisterStates(D15-D12)"=w337, "NI-845x Config for I2C (in)"=w338) -> ("error out"=w334:errorcluster, "NI-845x Config for I2C (out)"=w336:T13)  [unwired: 5 in]
        n93 = call "AD5933_SetStatus (NI-845x I2C)(SubVI).vi"("error in"=w334, "ConfigRegister (0x80)"=w321, "ControlRegisterStates(D15-D12)"=w335, "NI-845x Config for I2C (in)"=w336) -> ("error out"=w333:errorcluster, "NI-845x Config for I2C (out)"=w332:T13)  [unwired: 5 in]
        n94 = Get Date/Time In Seconds() -> (seconds since 1Jan1904=w312:timestamp)
        n95 = call "AD5933_ReadFrequencySweepValues (NI-845x I2C)(SubVI).vi"("error in"=w333, "ConfigRegister (0x80)"=w321, "NI-845x Config for I2C (in)"=w332) -> ("error out"=w318:errorcluster, "I Array"=w317:i16[], "R Array"=w319:i16[], "NI-845x Config for I2C (out)"=w330:T13)  [unwired: 4 in]
        n96 = call "AD5933_SetStatus (NI-845x I2C)(SubVI).vi"("error in"=w318, "ConfigRegister (0x80)"=w321, "ControlRegisterStates(D15-D12)"=w329, "NI-845x Config for I2C (in)"=w330) -> ("error out"=w310:errorcluster, "NI-845x Config for I2C (out)"=w328:T13)  [unwired: 5 in]
        n97 = Bundle By Name(cluster=w306, "Temperature"=w320, "R Array"=w319, "I Array"=w317, "Measurement Time"=w312) -> (w316:T2)
      }
      frame "Proceed Measurement and Wait" {
        w352 = FALSE ("Measurement Indicator")
        n98 = global read "MeasurementCluster.vi" "MeasurementCluster"() -> (w357:T11)
        n99 = Unbundle By Name(w357) -> ("Time Array"=w359:dbl[], "Impedance Matrix"=w363:dbl[][], "Phase Matrix"=w362:dbl[][], "Temperature Array"=w354:dbl[])
        n100 = Unbundle By Name(w350) -> ("Temperature"=w340:dbl, "Measurement Time"=w372:timestamp)
        n101 = Unbundle By Name(w366) -> ("Frequencies"=w351:dbl[])
        n102 = Unbundle By Name(w366) -> ("SaveMeas"=w378:bool, "refnum out"=w373:refnum<file>, "Frequencies"=w356:dbl[], "Sampling Rate [s]"=w371:dbl)
        n103 = Unbundle By Name(w375) -> ("Start Time"=w374:timestamp)
        n104 = call "AD5933_ImpedanceConversion (SubVI).vi"("Measurement Raw Data"=w350) -> ("Phase"=w341:dbl[], "Impedance"=w342:dbl[], "Imaginary Part"=w343:dbl[], "Real Part"=w344:dbl[], "Temperature"=w348:dbl)
        n105 = expression code="(x/pi)*180.0" "radians to degrees"(w341) -> (w349:dbl[])
        n106 = Subtract(x=w372, y=w374) -> (x-y=w358:dbl)
        n107 = Build Array (concatenate)(w359, w358) -> (w355:dbl[])
        n108 = Build Array (concatenate)(w363, w342) -> (w365:dbl[][])
        n109 = Build Array (concatenate)(w362, w341) -> (w364:dbl[][])
        n110 = Build Array (concatenate)(w354, w348) -> (w353:dbl[])
        n111 = case shown="True" w378 {
          tunnel: w373 -> [_ w397]
          tunnel: w358 -> [_ w401]
          tunnel: w342 -> [_ w400]
          tunnel: w341 -> [_ w398]
          tunnel: w340 -> [_ w399]
          frame False {
          }
          frame True {
            n112 = call "Save Data (SubVI).vi"("Time"=w401, "Impedance"=w400, "Phase"=w398, "Temperature"=w399, "Byte Stream File in"=w397) -> ()  [unwired: 1 in, 1 out]
          }
        }
        n113 = while {
          tunnel: w372 -> [w395]
          tunnel: w371 -> [w394]
          tunnel: ["Stop Measurement"] -> w370
          tunnel: w365 -> [w385]
          tunnel: w364 -> [w386]
          tunnel: w356 -> [w382]
          tunnel: w355 -> [w381]
          stop <- w393 stop-if-true
          n114 = Get Date/Time In Seconds() -> (seconds since 1Jan1904=w390:timestamp)
          n115 = Add(x=w395, y=w394) -> (x+y=w391:timestamp)
          n116 = Subtract(x=w391, y=w390) -> (x-y=w388:dbl)
          "Next measurement" <- w388
          n117 = Less Or Equal To 0?(x=w388) -> (x <= 0?=w389:bool)
          n118 = Search 1D Array(1D array=w382, element="Frequency [Hz]") -> (index of element=w380:i32)  [unwired: 1 in]
          n119 = Index Array(array=w385, index (col)=w380) -> (element=w384:dbl[])  [unwired: 1 in]
          n120 = Index Array(array=w386, index (col)=w380) -> (element=w383:dbl[])  [unwired: 1 in]
          n121 = Build Cluster Array(w381, w384, w383) -> (→"|Z|,phi vs Time":T15)
          n122 = Or(x=w389, y="Stop Measurement") -> (x .or. y?=w393:bool)
          n123 = Wait (ms)(milliseconds to wait=u32 200 ("millisecond multiple")) -> ()  [unwired: 1 out]
        }
        n124 = Build Cluster Array(w351, w342, w349) -> (→"|Z|,phi vs Frequency":cluster{dbl, "Impedance":dbl, "Phase":dbl}[])
        n125 = Build Cluster Array(w355, w353) -> (→"Temperature vs Time":cluster{"x-y":dbl, "Temperature":dbl}[])
        n126 = Build Cluster Array(w351, w344, w343) -> (→"Real,Imag vs Frequency":cluster{dbl, dbl, dbl}[])
        n127 = Bundle By Name(cluster=w357, "Time Array"=w355, "Impedance Matrix"=w365, "Phase Matrix"=w364, "Temperature Array"=w353) -> (w361:T11)
        n128 = local write "Measurement Indicator"(w352) -> ()
        n129 = property on="Measurement Indicator" class="Bool"("Visible"=w352) -> ()  [unwired: 2 in, 2 out]
        n130 = global write "MeasurementCluster.vi" "MeasurementCluster"(w361) -> ()
        n131 = Select(t=StateMachnie_States."Stop Measurement", s=w370, f=StateMachnie_States."Do Measurement") -> (s? t:f=w367:T8)
      }
      frame "Stop Measurement" {
        w402 = T9."Enabled" ("Disabled")
        n132 = Unbundle By Name(w409) -> ("SaveMeas"=w406:bool, "refnum out"=w413:refnum<file>)
        n133 = case shown="True" w406 {
          tunnel: w413 -> [_ w415]
          tunnel: w412 -> [w414 w416]
          tunnel: [w414 w417] -> w403
          frame False {
          }
          frame True {
            n134 = Close File(refnum=w415, error in=w416) -> (error out=w417:errorcluster)  [unwired: 1 out]
          }
        }
        n135 = property on="Calibrate" class="Bool"("DisabledEnum"=w402) -> ()  [unwired: 2 in, 2 out]
        n136 = property on="Set Configuration" class="Bool"("DisabledEnum"=w402) -> ()  [unwired: 2 in, 2 out]
        n137 = property on="Start" class="Bool"("DisabledEnum"=w402) -> ()  [unwired: 2 in, 2 out]
        n138 = property on="Stop Measurement" class="Bool"("DisabledEnum"=T9."Disabled and Grayed Out" ("Disabled")) -> ()  [unwired: 2 in, 2 out]
      }
    }
    n139 = call <vilib>:"Simple Error Handler.vi"("error in (no error)"=w12) -> ("error out"=w13:errorcluster)  [unwired: 4 in, 4 out]
    n140 = call <vilib>:"Clear Errors.vi"("error in (no error)"=w13) -> ("error out"=w11:errorcluster)  [unwired: 5 in, 1 out]
  }
  n141 = disable-structure shown="RUN_TIME_ENGINE==True" {
    disable-tunnel: w2 -> [_ _]
    frame condition #0 (active) {
    }
    frame condition #1 {
      # "Call Quit LabVIEW if running as a built application."
      n142 = Quit LabVIEW() -> ()  [unwired: 1 in]
    }
  }
  "Measurement Indicator" <- w1
